vi "路径.vi"(11 "应用程序输入":refnum<vi>) -> (3 "stripped path":path)   [LabVIEW 2012]
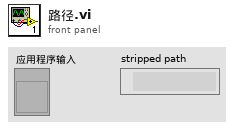
[diagram p1: front panel]
types:
  T1 = enum32{"invalid app kind", "Development System", "Run Time System", "Student Edition", "Embedded LabVIEW", "Evaluation", "Custom"}
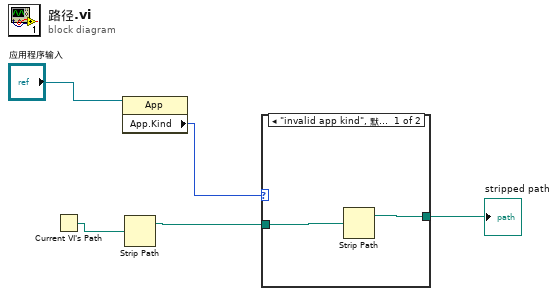
[diagram p0: block diagram]
diagram:
  n1 = Current VI's Path() -> (path=w2:path)
  n2 = property class="App"(reference="应用程序输入") -> ("App.Kind"=w3:T1)  [unwired: 1 in, 2 out]
  n3 = Strip Path(path=w2) -> (stripped path=w4:path)  [unwired: 1 out]
  n4 = case shown="\"invalid app kind\", 默认" w3 {
    tunnel: w4 -> [w7 w8]
    tunnel: [w6 w8] -> w5
    frame "invalid app kind", Default {
      n5 = Strip Path(path=w7) -> (stripped path=w6:path)  [unwired: 1 out]
    }
    frame "Development System" {
    }
  }
  "stripped path" <- w5
